vi "PCB_ElectricalTests.vi"() -> ()   [LabVIEW 2015]
panel:
  in  "New Session":bool
  in  "Stop Button":bool
  in  "Tab Control":T1(tab)
  in  "DONE WITH PCB NAMING?":bool
  in  "DONE WITH BOTH SIDES?":bool
  in  "Punto 1 (MOhm)":string
  in  "Punto 2 (MOhm)":string
  in  "Punto 3 (MOhm)":string
  in  "Punto 4 (MOhm)":string
  in  "Punto 5 (MOhm)":string
  in  "PCB NAME (e.g SE1004)":string
  in  "Punto 1 (MOhm)":string
  in  "Punto 2 (MOhm)":string
  in  "Punto 3 (MOhm)":string
  in  "Punto 4 (MOhm)":string
  in  "Punto 5 (MOhm)":string
  in  "Comment":string
  in  "Punto 9 (MOhm)":string
  in  "Punto 8 (MOhm)":string
  in  "Punto 7 (MOhm)":string
  in  "Punto 6 (MOhm)":string
  in  "Punto 9 (MOhm)":string
  in  "Punto 8 (MOhm)":string
  in  "Punto 7 (MOhm)":string
  in  "Punto 6 (MOhm)":string
  in  "Punto 1 (MOhm)":string
  in  "Punto 2 (MOhm)":string
  in  "Punto 3 (MOhm)":string
  in  "Punto 4 (MOhm)":string
  in  "Punto 5 (MOhm)":string
  in  "Punto 1 (MOhm)":string
  in  "Punto 2 (MOhm)":string
  in  "Punto 3 (MOhm)":string
  in  "Punto 4 (MOhm)":string
  in  "Punto 5 (MOhm)":string
  in  "DONE WITH BOTH SIDES?":bool
  in  "Comment":string
  in  "DX (GOhm)":string
  in  "SX (GOhm)":string
  in  "DONE WITH BOTH SIDES?":bool
  in  "Comment":string
  in  "Meas. 4 (GOhm)":string
  in  "Meas. 3 (GOhm)":string
  in  "DONE WITH BOTH SIDES?":bool
  in  "Meas. 2 (GOhm)":string
  in  "Meas. 1 (GOhm)":string
  in  "Comment":string
  # "In this test the resistance of the resistive strips is measured. \nThe measurement is performed between the the resistive strips and the HV.\nThe measurement points are on the borders of the pillar region and the restistive strip contact is achieved through the use of the plexiglass tool probes.\nTools needed: \n- Plexiglass tool with probes\n- Multimeter\n- Two cables with banana plugs\n\nInstructions:\n- Place the electrical tool on one of the PCB sides\n- Connect the first cable on one multimeter pole on one end and on the HV probe on the other\n- Connect the second cable on the other multimeter pole on one end and on one of the 5 resistive strip probes of the other\n- Switch on the multimeter, switch it to the resistance measurement (Ohm) and place it on the table\n- Wait a few seconds until the measurement is stabilized. You should see a value of a few MOhm"
  # "Cu strips"
  # "Silverline"
  # "1"
  # "1"
  # "SX"
  # "SX"
  # "DX"
  # "2"
  # "2"
  # "HV"
  # "HV"
  # "3"
  # "3"
  # "4"
  # "4"
  # "Cu strips"
  # "DX"
  # "5"
  # "5"
  # "In this test the resistance of the resistive strips is measured. \nThe measurement is performed between the resistive strips and the HV.\nThe measurement points are all over the main pillar region and the restistive strip contact is achieved through the use of a single probe (batticarne).\nTools needed: \n- Plexiglass tool with probes\n- Batticarne, plasticized card for the precise positioning of the tool\n- Multimeter\n- Two cables with banana plugs\n\nInstructions:\n- Place the electrical tool on one of the PCB sides\n- Place the plasticized card on the main pillar region in such a way that it is parallel to the PCB sides and close to the plexiglass tool\n- Place the batticarne on point 1 rotated such that the line designed on it and the line of the card hole coincide\n- Connect the first cable on one multimeter pole on one end and on the HV probe on the other\n- Connect the second cable on the other multimeter pole on one end and on the probe of the batticarne\n- Switch on the multimeter, switch it to the resistance measurement (Ohm) and place it on the table\n- Wait a few seconds until the measurement is stabilized. A value of a few MOhm should be obtained."
  # "1"
  # "4"
  # "4"
  # "1"
  # "SX"
  # "DX"
  # "2"
  # "5"
  # "5"
  # "2"
  # "SX"
  # "DX"
  # "3"
  # "6"
  # "6"
  # "3"
  # "In this test the isolation of the silverline due to the coverlay is measured. \nThe measurement is performed between the silverline and the HV.\nThe measurement points are the probe (either of the two) of the silverline and the HV probe.\nThis is a HV measurement so be very careful to NOT touch the board while measuring!\nTools needed: \n- Plexiglass tool with probes\n- Megger\n- Two HV cables with banana plugs\n\nInstructions:\n- Place the electrical tool on one of the PCB sides\n- Open the Megger box and connect the HV cables on the + and - inputs\n- Connect the other end of one of the HV cables on the silverline probe\n- Connect the other end of the second HV on the HV probe\n- MAKE SURE THE HV CABLES ARE CONNECTED TO THE RIGHT PROBES!!! MAKE SURE THERE ARE NO OBJECTS ON THE PCB!\n- Switch on the Megger and set it to 1000V for 2 minutes\n- Move away from the PCB!\n- Start the measurement by keeping pressed the red button until you hear a clicking sound\n- Wait until the measurement ends (Megger light will switch off, and you will hear the clicking sound again)"
  # "Here you should see a value of above 100 GOhm."
  # "In this test the isolation of the Cu strips from the resistive strips due to the kapton layer is measured. \nThe measurement is performed between the HV and Cu strips.\nThe measurement points are the HV probe (or the batticarne probe) and the Cu strip probe.\nThis is a HV measurement so be very careful to NOT touch the board while measuring!\nTools needed: \n- Plexiglass tool with probes\n- Megger\n- Batticarne\n- Two HV cables with banana plugs\n\nInstructions:\nSince the resistive strips are cut in the middle of the PCB (left from right) and the Cu strips are divided into two sides (up and down), there \nare 4 measurements to be performed.\n- Measurement 1: HV probe vs. Cu strips (top right PCB part)\n- Measurement 2: Batticarne probe vs. Cu strips (top left PCB part)\n- Measurement 3: HV probe vs. Cu strips (bottom left PCB part)\n- Measurement 4: Batticarne probe vs. Cu strips (bottom right PCB part)"
  # "Here you should see a value of above 10 GOhm."
  # "SX"
  # "DX"
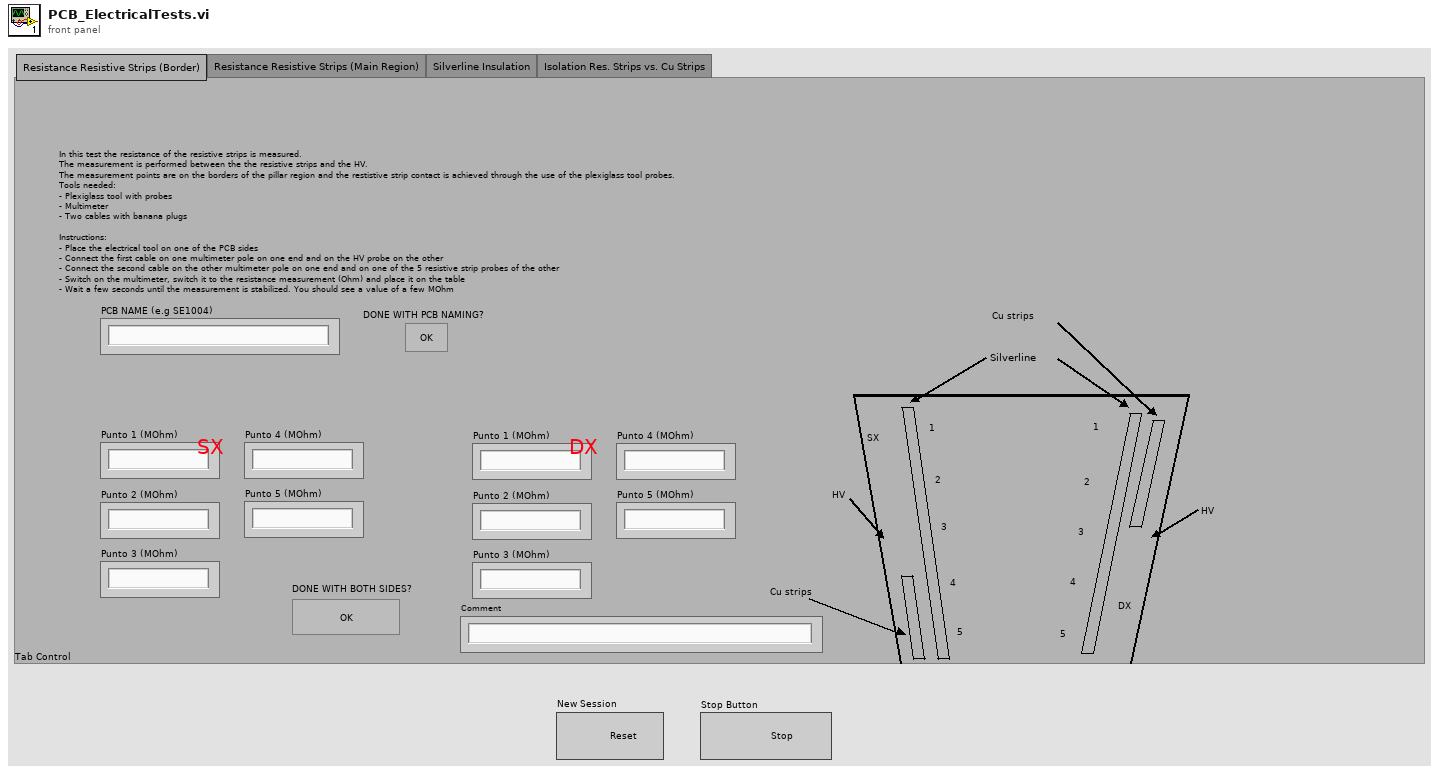
[diagram p1: front panel]
types:
  T1 = enum32{"Resistance Resistive Strips (Border)", "Resistance Resistive Strips (Main Region)", "Silverline Insulation", "Isolation Res. Strips vs. Cu Strips"}
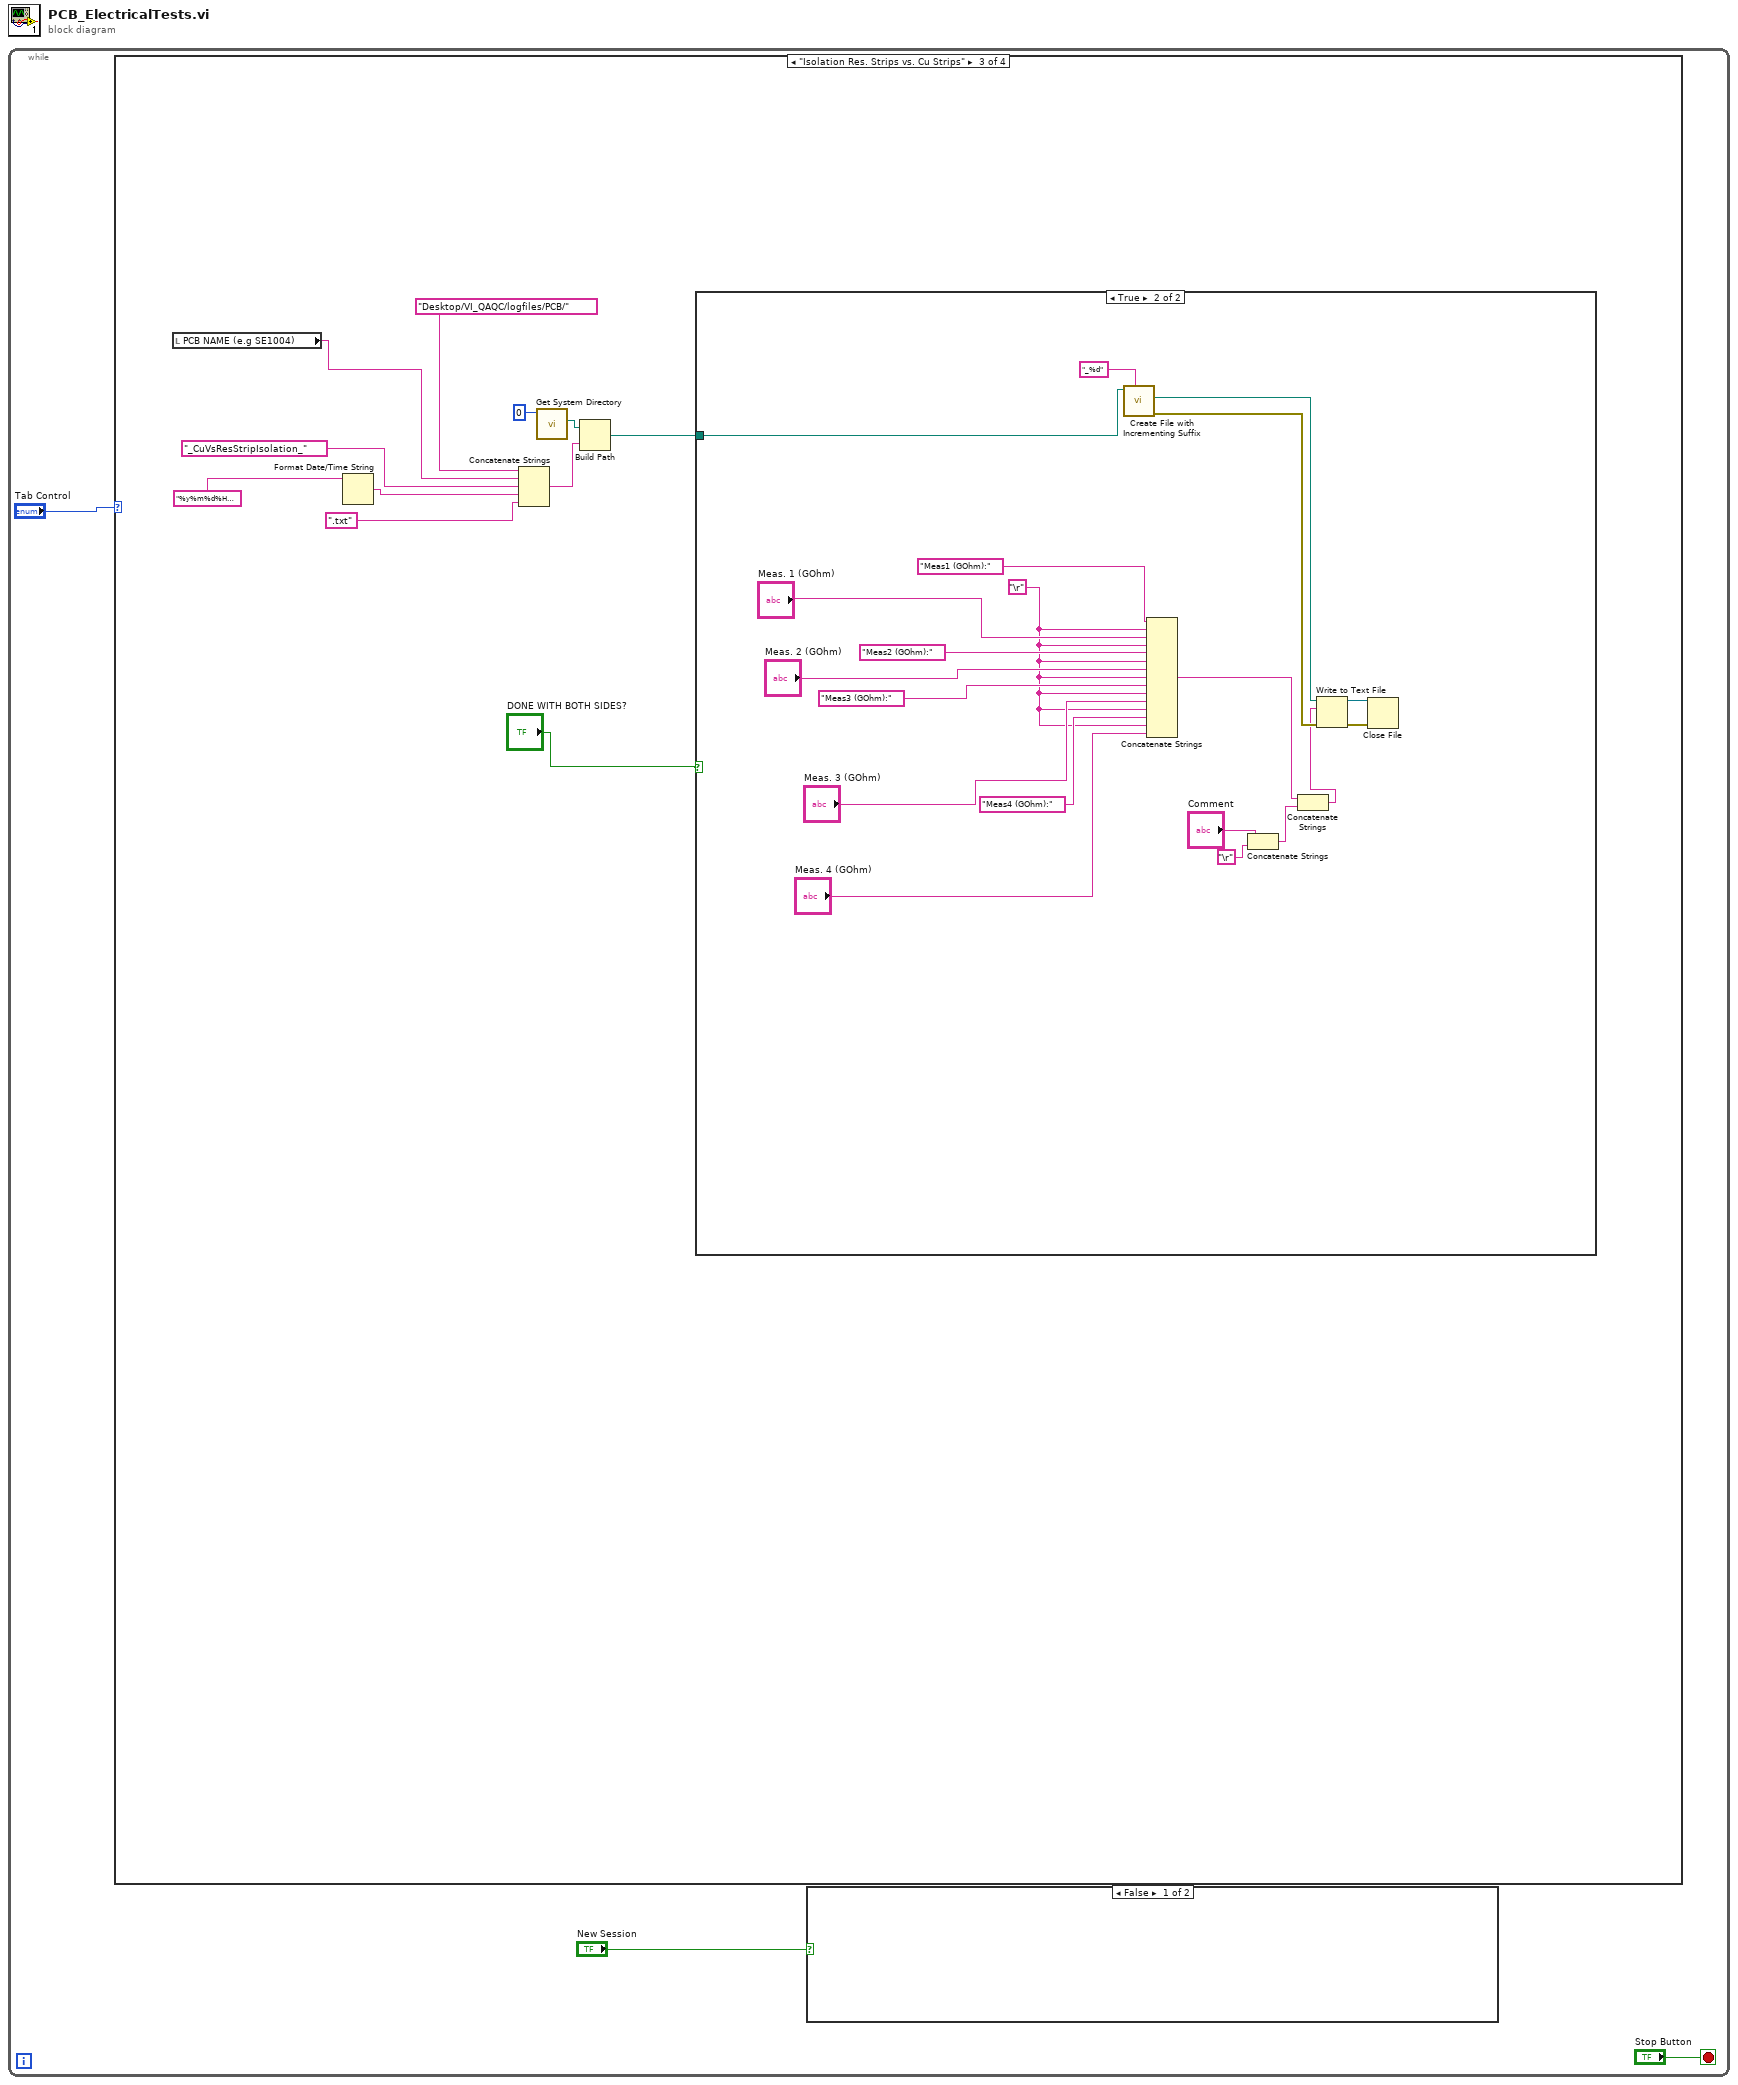
[diagram p0: block diagram]
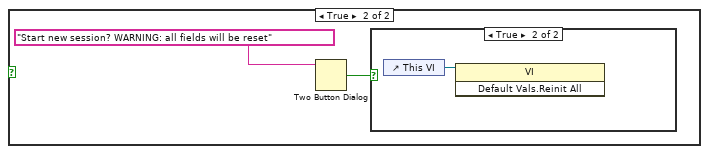
[diagram p2: hidden frame]
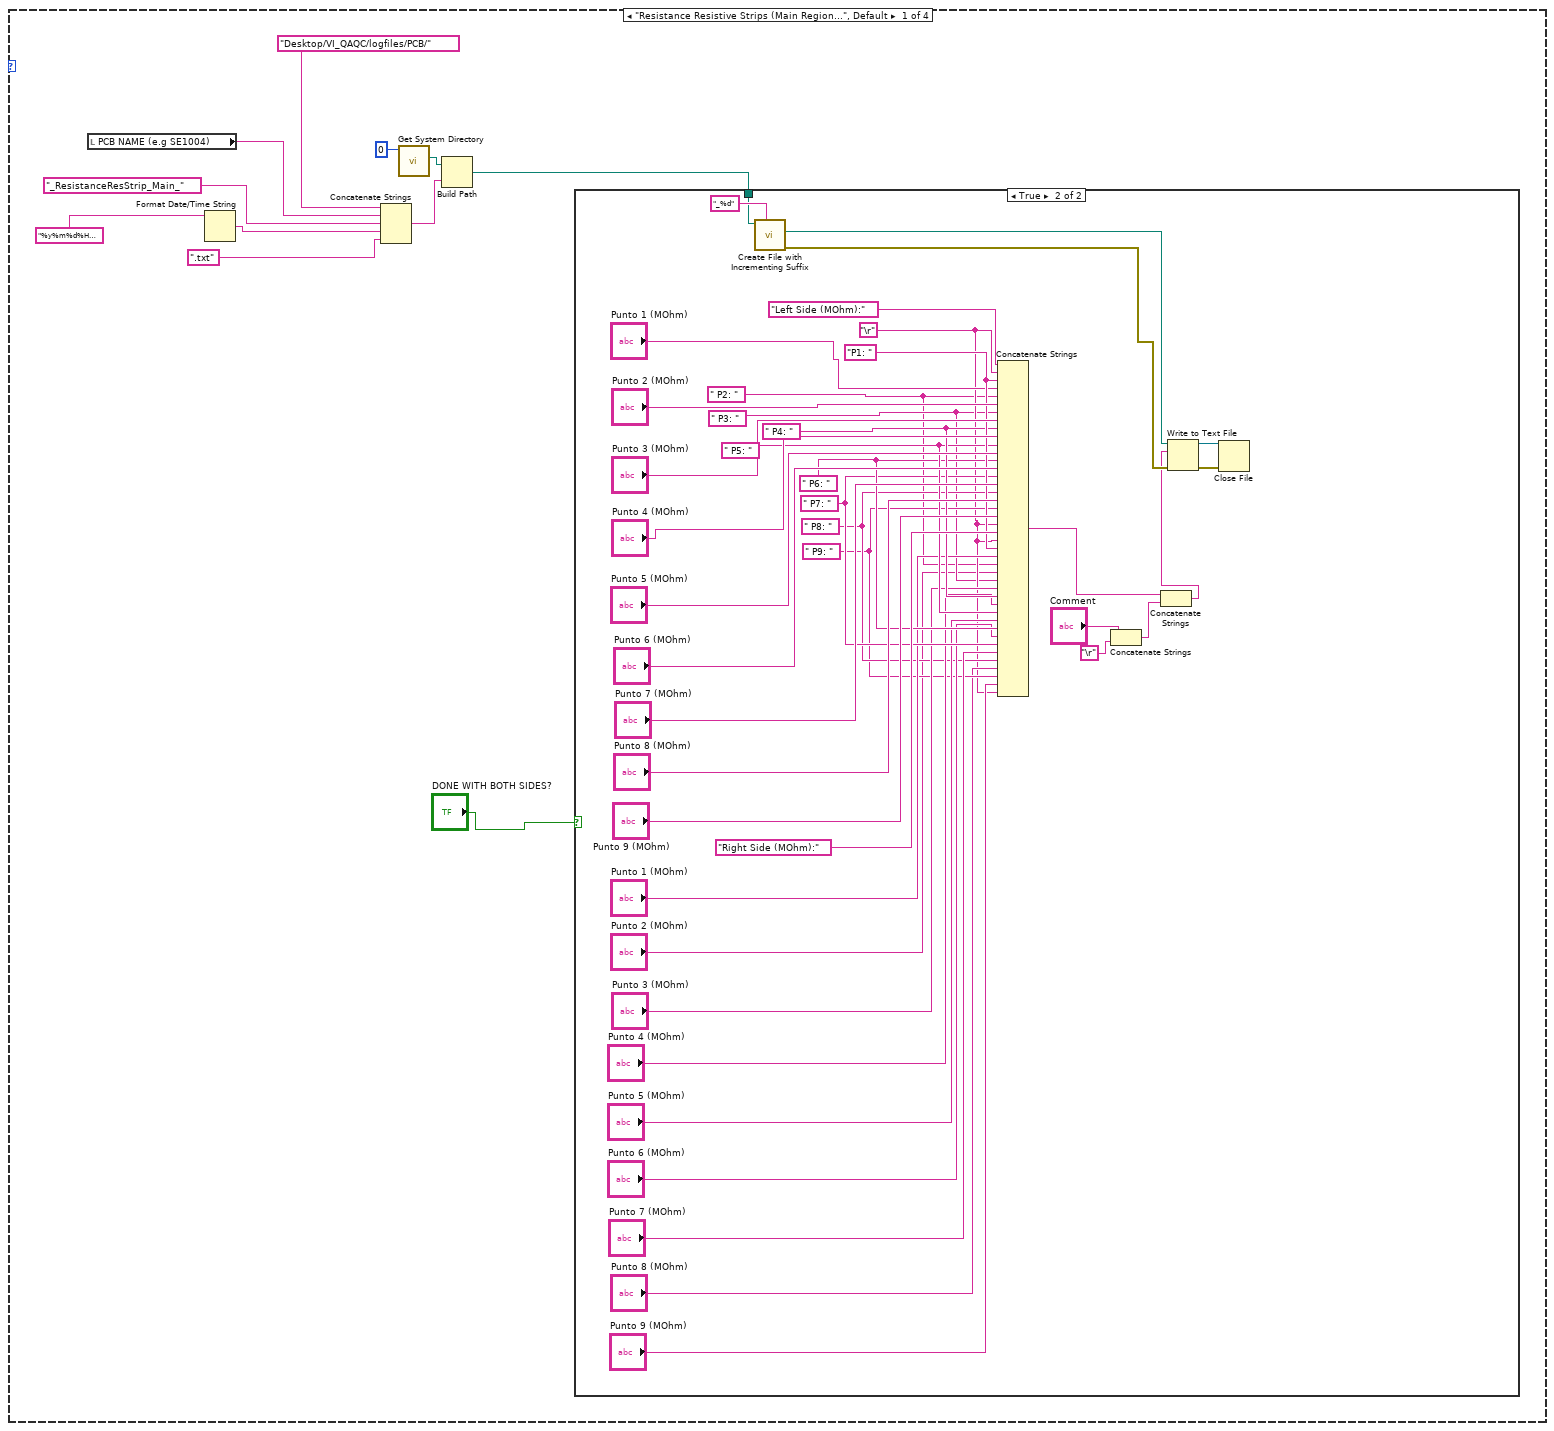
[diagram p4: hidden frame]
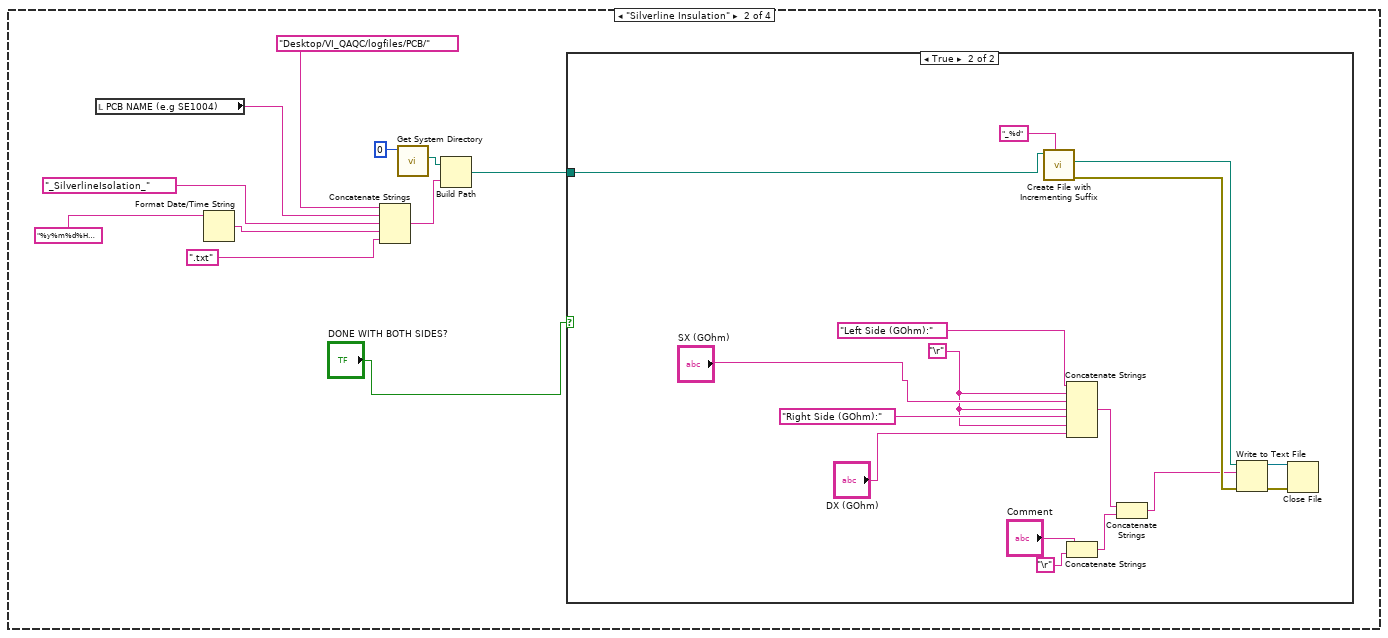
[diagram p6: hidden frame]
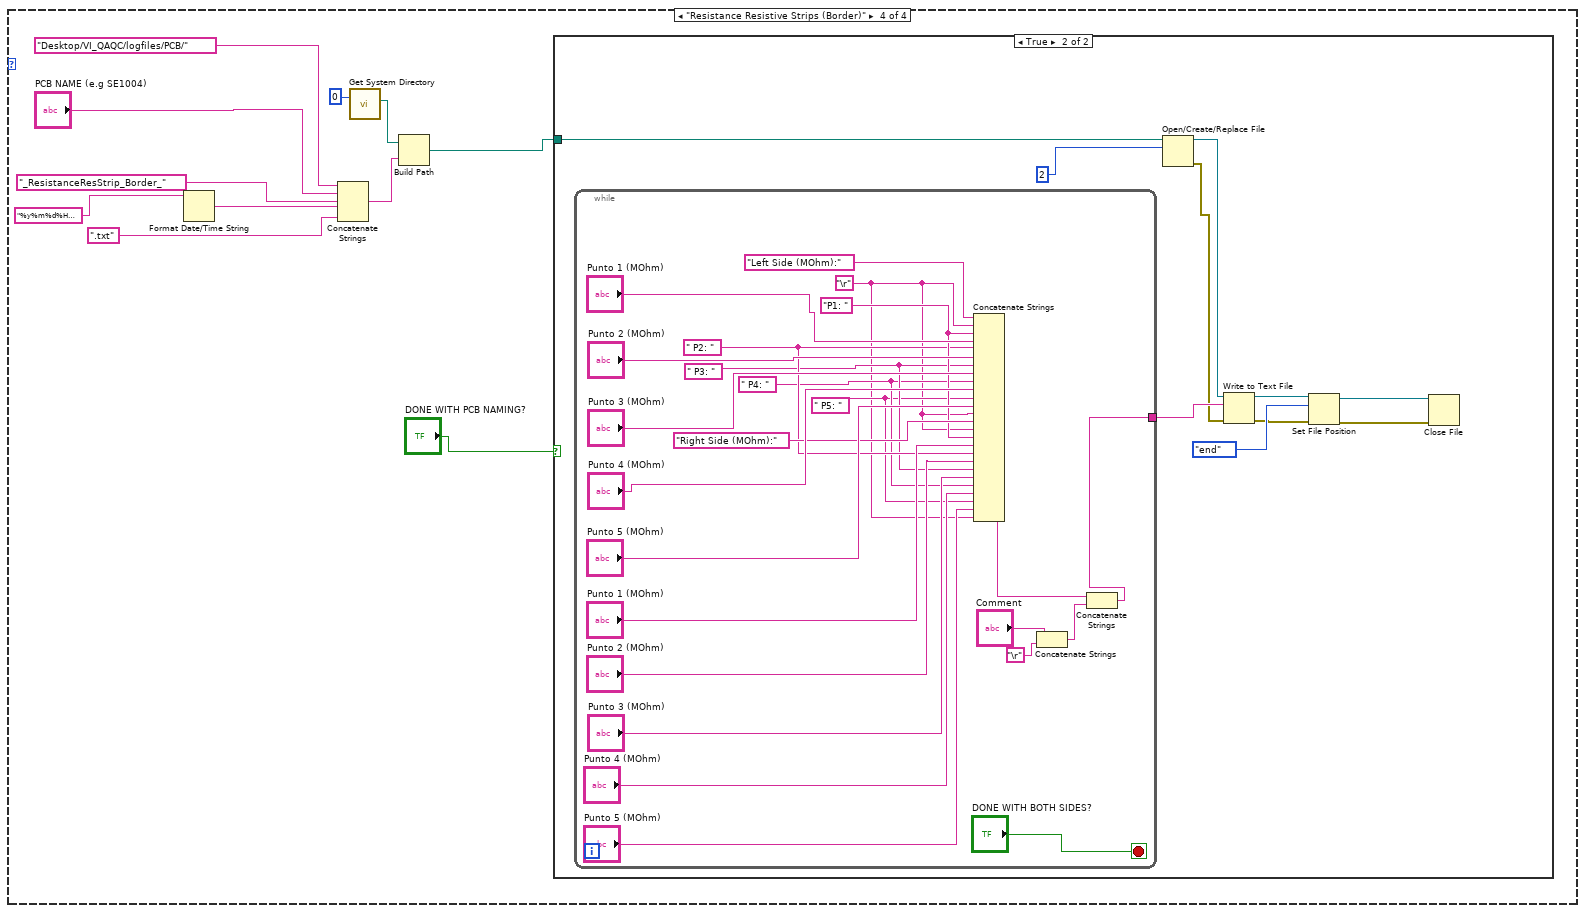
[diagram p9: hidden frame]
diagram:
  n1 = while {
    stop <- "Stop Button" stop-if-true
    n2 = case shown="\"Isolation Res. Strips vs. Cu Strips\"" "Tab Control" {
      frame "Resistance Resistive Strips (Main Region)", Default {
        n3 = local read "PCB NAME (e.g SE1004)"() -> (w9:string)
        n4 = Format Date/Time String(time format string (%c)="%y%m%d%H%M") -> (date/time string=w10:string)  [unwired: 2 in]
        n5 = Concatenate Strings("Desktop/VI_QAQC/logfiles/PCB/", w9, "_ResistanceResStrip_Main_", w10, ".txt") -> (w15:string)
        n6 = call <vilib>:"Get System Directory.vi"("system directory type"=0) -> ("system directory"=w16:path)  [unwired: 10 in]
        n7 = Build Path(base path=w16, name or relative path=w15) -> (appended path=w7:path)
        n8 = case shown="True" "DONE WITH BOTH SIDES?" {
          tunnel: w7 -> [_ w28]
          frame False {
          }
          frame True {
            w33 = " P9: "
            w34 = " P8: "
            w41 = " P7: "
            w42 = " P6: "
            w43 = " P5: "
            w44 = " P4: "
            w25 = " P3: "
            w23 = " P2: "
            w46 = "P1: "
            w30 = "\r"
            n9 = call <vilib>:"Create File with Incrementing Suffix.vi"("format string (\" (%d)\")"="_%d" ("format string (\" (%d)\")"), "file path"=w28) -> ("error out"=w27:errorcluster, "actual path"=w26:path)  [unwired: 7 in, 1 out]
            n10 = Concatenate Strings("Left Side (MOhm):", w30, w46, "Punto 1 (MOhm)", w23, "Punto 2 (MOhm)", w25, "Punto 3 (MOhm)", w44, "Punto 4 (MOhm)", w43, "Punto 5 (MOhm)", w42, "Punto 6 (MOhm)", w41, "Punto 7 (MOhm)", w34, "Punto 8 (MOhm)", w33, "Punto 9 (MOhm)", w30, "Right Side (MOhm):", w30, w46, "Punto 1 (MOhm)", w23, "Punto 2 (MOhm)", w25, "Punto 3 (MOhm)", w44, "Punto 4 (MOhm)", w43, "Punto 5 (MOhm)", w42, "Punto 6 (MOhm)", w41, "Punto 7 (MOhm)", w34, "Punto 8 (MOhm)", w33, "Punto 9 (MOhm)", w30) -> (w22:string)
            n11 = Concatenate Strings("Comment", "\r") -> (w20:string)
            n12 = Concatenate Strings(w22, w20) -> (w21:string)
            n13 = Write to Text File(file (use dialog)=w26, text=w21, error in=w27) -> (refnum out=w57:refnum<file>, error out=w58:errorcluster)  [unwired: 1 in, 1 out]
            n14 = Close File(refnum=w57, error in=w58) -> ()  [unwired: 2 out]
          }
        }
      }
      frame "Silverline Insulation" {
        n15 = local read "PCB NAME (e.g SE1004)"() -> (w60:string)
        n16 = Format Date/Time String(time format string (%c)="%y%m%d%H%M") -> (date/time string=w61:string)  [unwired: 2 in]
        n17 = Concatenate Strings("Desktop/VI_QAQC/logfiles/PCB/", w60, "_SilverlineIsolation_", w61, ".txt") -> (w67:string)
        n18 = call <vilib>:"Get System Directory.vi"("system directory type"=0) -> ("system directory"=w68:path)  [unwired: 10 in]
        n19 = Build Path(base path=w68, name or relative path=w67) -> (appended path=w66:path)
        n20 = case shown="True" "DONE WITH BOTH SIDES?" {
          tunnel: w66 -> [_ w82]
          frame False {
          }
          frame True {
            w76 = "\r"
            n21 = call <vilib>:"Create File with Incrementing Suffix.vi"("format string (\" (%d)\")"="_%d" ("format string (\" (%d)\")"), "file path"=w82) -> ("error out"=w80:errorcluster, "actual path"=w81:path)  [unwired: 7 in, 1 out]
            n22 = Concatenate Strings("Left Side (GOhm):", w76, "SX (GOhm)", w76, "Right Side (GOhm):", w76, "DX (GOhm)") -> (w71:string)
            n23 = Concatenate Strings("Comment", "\r") -> (w74:string)
            n24 = Concatenate Strings(w71, w74) -> (w70:string)
            n25 = Write to Text File(file (use dialog)=w81, text=w70, error in=w80) -> (refnum out=w84:refnum<file>, error out=w85:errorcluster)  [unwired: 1 in, 1 out]
            n26 = Close File(refnum=w84, error in=w85) -> ()  [unwired: 2 out]
          }
        }
      }
      frame "Isolation Res. Strips vs. Cu Strips" {
        n27 = local read "PCB NAME (e.g SE1004)"() -> (w87:string)
        n28 = Format Date/Time String(time format string (%c)="%y%m%d%H%M") -> (date/time string=w88:string)  [unwired: 2 in]
        n29 = Concatenate Strings("Desktop/VI_QAQC/logfiles/PCB/", w87, "_CuVsResStripIsolation_", w88, ".txt") -> (w94:string)
        n30 = call <vilib>:"Get System Directory.vi"("system directory type"=0) -> ("system directory"=w95:path)  [unwired: 10 in]
        n31 = Build Path(base path=w95, name or relative path=w94) -> (appended path=w93:path)
        n32 = case shown="True" "DONE WITH BOTH SIDES?" {
          tunnel: w93 -> [_ w113]
          frame False {
          }
          frame True {
            w103 = "\r"
            n33 = call <vilib>:"Create File with Incrementing Suffix.vi"("format string (\" (%d)\")"="_%d" ("format string (\" (%d)\")"), "file path"=w113) -> ("error out"=w111:errorcluster, "actual path"=w112:path)  [unwired: 7 in, 1 out]
            n34 = Concatenate Strings("Meas1 (GOhm):", w103, "Meas. 1 (GOhm)", w103, "Meas2 (GOhm):", w103, "Meas. 2 (GOhm)", w103, "Meas3 (GOhm):", w103, "Meas. 3 (GOhm)", w103, "Meas4 (GOhm):", w103, "Meas. 4 (GOhm)") -> (w98:string)
            n35 = Concatenate Strings("Comment", "\r") -> (w101:string)
            n36 = Concatenate Strings(w98, w101) -> (w97:string)
            n37 = Write to Text File(file (use dialog)=w112, text=w97, error in=w111) -> (refnum out=w115:refnum<file>, error out=w116:errorcluster)  [unwired: 1 in, 1 out]
            n38 = Close File(refnum=w115, error in=w116) -> ()  [unwired: 2 out]
          }
        }
      }
      frame "Resistance Resistive Strips (Border)" {
        n39 = Format Date/Time String(time format string (%c)="%y%m%d%H%M") -> (date/time string=w120:string)  [unwired: 2 in]
        n40 = Concatenate Strings("Desktop/VI_QAQC/logfiles/PCB/", "PCB NAME (e.g SE1004)", "_ResistanceResStrip_Border_", w120, ".txt") -> (w125:string)
        n41 = call <vilib>:"Get System Directory.vi"("system directory type"=0) -> ("system directory"=w126:path)  [unwired: 10 in]
        n42 = Build Path(base path=w126, name or relative path=w125) -> (appended path=w119:path)
        n43 = case shown="True" "DONE WITH PCB NAMING?" {
          tunnel: w119 -> [_ w136]
          frame False {
          }
          frame True {
            n44 = while {
              tunnel: [w138] -> w137
              stop <- "DONE WITH BOTH SIDES?" stop-if-true
              w146 = " P5: "
              w148 = " P4: "
              w150 = " P3: "
              w152 = " P2: "
              w154 = "P1: "
              w144 = "\r"
              n45 = Concatenate Strings("Left Side (MOhm):", w144, w154, "Punto 1 (MOhm)", w152, "Punto 2 (MOhm)", w150, "Punto 3 (MOhm)", w148, "Punto 4 (MOhm)", w146, "Punto 5 (MOhm)", w144, "Right Side (MOhm):", w144, w154, "Punto 1 (MOhm)", w152, "Punto 2 (MOhm)", w150, "Punto 3 (MOhm)", w148, "Punto 4 (MOhm)", w146, "Punto 5 (MOhm)", w144) -> (w139:string)
              n46 = Concatenate Strings("Comment", "\r") -> (w142:string)
              n47 = Concatenate Strings(w139, w142) -> (w138:string)
            }
            n48 = Open/Create/Replace File(file path (use dialog)=w136, operation (0:open)=2) -> (refnum out=w134:refnum<file>, error out=w135:errorcluster)  [unwired: 4 in, 1 out]
            n49 = Write to Text File(file (use dialog)=w134, text=w137, error in=w135) -> (refnum out=w131:refnum<file>, error out=w129:errorcluster)  [unwired: 1 in, 1 out]
            n50 = Set File Position(offset (in bytes) (0)=enum16{"end"}."end", refnum=w131, error in=w129) -> (refnum out=w130:refnum<file>, error out=w128:errorcluster)  [unwired: 1 in]
            n51 = Close File(refnum=w130, error in=w128) -> ()  [unwired: 2 out]
          }
        }
      }
    }
    n52 = case shown="False" "New Session" {
      frame False {
      }
      frame True {
        n53 = Two Button Dialog(message="Start new session? WARNING: all fields will be reset") -> (T button?=w4:bool)  [unwired: 2 in]
        n54 = case shown="True" w4 {
          frame False {
          }
          frame True {
            n55 = control-ref of="This VI"() -> (w6:refnum<vi>)
            n56 = invoke class="VI" method="Default Vals.Reinit All"(reference=w6) -> ()  [unwired: 2 in, 3 out]
          }
        }
      }
    }
  }
